vi "Day 6.2 - group generations.vi"(7 "Generations":i32=80, 11 "input":string[](array[string])) -> (3 "output":u64)   [LabVIEW 2021]
panel:
  out "Waveform Graph":u64[][](graph)
  out "Array":u64[](array[numeric])
  # "e"
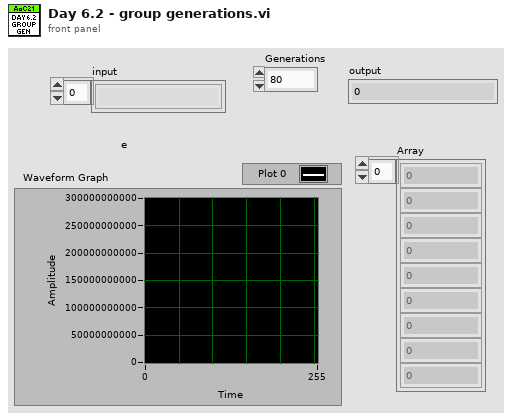
[diagram p1: front panel]
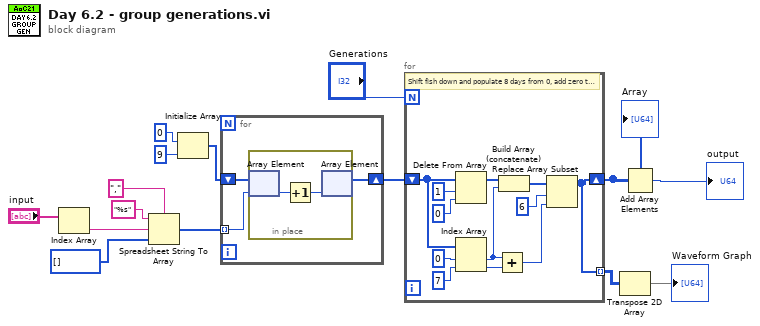
[diagram p0: block diagram]
diagram:
  n1 = Index Array(array="input") -> (element=w14:string)  [unwired: 1 in]
  n2 = Spreadsheet String To Array(delimiter (Tab)=",", format string="%s", spreadsheet string=w14, array type (2D Dbl)=i32[] []) -> (array=w8:i32[])
  n3 = Initialize Array(u64 0, 9 ("dimension size")) -> (w5:u64[])
  n4 = for {
    tunnel: w8 -> [w17] mode=indexing
    shift-right: [w16] -> w6
    shift-left: w5 -> [w18]
    n5 = in-place {
      n6 = in-place-array #1(w18, w17) -> (w20:u64)
      n7 = Increment(x=w20) -> (x+1=w19:u64)
      n8 = in-place-array #1(w19) -> (w16:u64[])  [unwired: 1 out]
    }
  }
  n9 = for {
    N: "Generations" -> [_]
    shift-right: [w21] -> w3
    shift-left: w6 -> [w30]
    tunnel: [w21] -> w2 mode=indexing
    # "Shift fish down and populate 8 days from 0, add zero to pos 6"
    n10 = Delete From Array(array=w30, length=1, index=0) -> (array with subset deleted=w27:u64[])  [unwired: 1 out]
    n11 = Index Array(array=w30, index #1=0 ("index"), index #2=7 ("index")) -> (element #1=w25:u64, element #2=w26:u64)
    n12 = Add(x=w25, y=w26) -> (x+y=w22:u64)
    n13 = Build Array (concatenate)(w27, w25) -> (w24:u64[])
    n14 = Replace Array Subset(array=w24, new element=w22, index=6) -> (w21:u64[])
  }
  "Array" <- w3
  n15 = Transpose 2D Array(2D array=w2) -> (transposed array=→"Waveform Graph":u64[][])
  n16 = Add Array Elements(numeric array=w3) -> (sum=→"output":u64)
